vi "fake_scope.vi"() -> ()   [LabVIEW 2013]
doc: "This example shows how to use autosetup and acquire a waveform on a single channel for acquiring waveforms in a loop until stopped by user."
uses:
  osc_channel.ctl
  Global.vi
panel:
  out "SQUID":string="2"
  in  "stop":bool
  in  "Tab Control":T1(tab)
  out "Saving":bool
  out "Waveform Data":waveform(dbl)[](graph)=[{"t0"=timestamp(0 s since 1904-01-01), "dt"=6e-09, "Y"=array[1000 elements]}, {"t0"=timestamp(0 s since 1904-01-01), "dt"=6e-09, "Y"=array[1000 elements]}]
  in  "Points":i32=1000
  out "dt":dbl=6e-09 format="%#_2e"
  out "Repeat":u32=16
  out "Manufacturer":string="Skynet"
  out "Model":string="T1000"
  in  "Record":bool[](array[boolean])=[TRUE, FALSE]
  out "Stats":T2(array[cluster])=[{"Min"=-0.9973419383523257, "t (min)"=4.686e-06, "Max"=1.093351892163248, "t (max)"=1.53e-06, "Range"=2.0906938305155736, "Mean"=0.058141922470583494, "Std"=0.7227490723476767}, {"Min"=-0.5, "t (min)"=3.6779999999999998e-06, "Max"=0.5, "t (max)"=4.44e-07, "Range"=1.0, "Mean"=0.021262229190316277, "Std"=0.4513064444152934}] {"t (min)" format="%#_6p"; "t (max)" format="%#_6p"}
  in  "Channels":T3[](array[typedef])=[{"channel name"="CHANNEL1", "probe attenuation"=1.0, "vertical offset"=0.0, "vertical range"=10.0, "vertical coupling"=1, "input impedance"=50.0}, {"channel name"="CHANNEL2", "probe attenuation"=1.0, "vertical offset"=0.0, "vertical range"=1.0, "vertical coupling"=1, "input impedance"=50.0}] {"input impedance" format="%#_13g"; "vertical coupling" items=["AC", "DC", "GND"]; "vertical range" format="%.3f"; "vertical offset" format="%.3f"; "probe attenuation" format="%.3f"}
  in  "wait (ms)":u32=500
  in  "Bin size":i16=1
  in  "sample":dbl=6e-06
  in  "amplitude":dbl=1.0 format="%#_13g"
  in  "noise":dbl=0.1 format="%#_13g"
  in  "frequency":dbl=1000000.0 format="%#_13g"
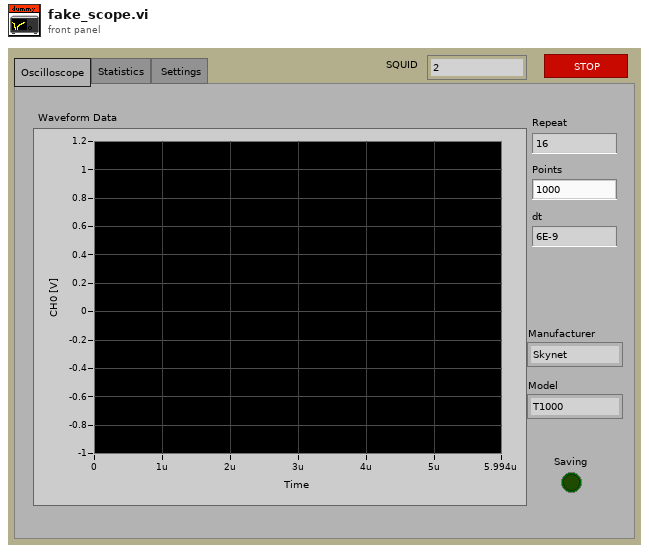
[diagram p1: front panel]
types:
  T1 = enum32{"Oscilloscope", "Statistics", " Settings"}
  T2 = cluster{"Min":dbl, "t (min)":dbl, "Max":dbl, "t (max)":dbl, "Range":dbl, "Mean":dbl, "Std":dbl}[]
  T3 = typedef "osc_channel.ctl" = cluster{"channel name":string, "probe attenuation":dbl, "vertical offset":dbl, "vertical range":dbl, "vertical coupling":i32, "input impedance":dbl}
  T4 = cluster{"Min":dbl, "t (min)":dbl, "Max":dbl, "t (max)":dbl, "Range":dbl, "Mean":dbl, "Std":dbl}
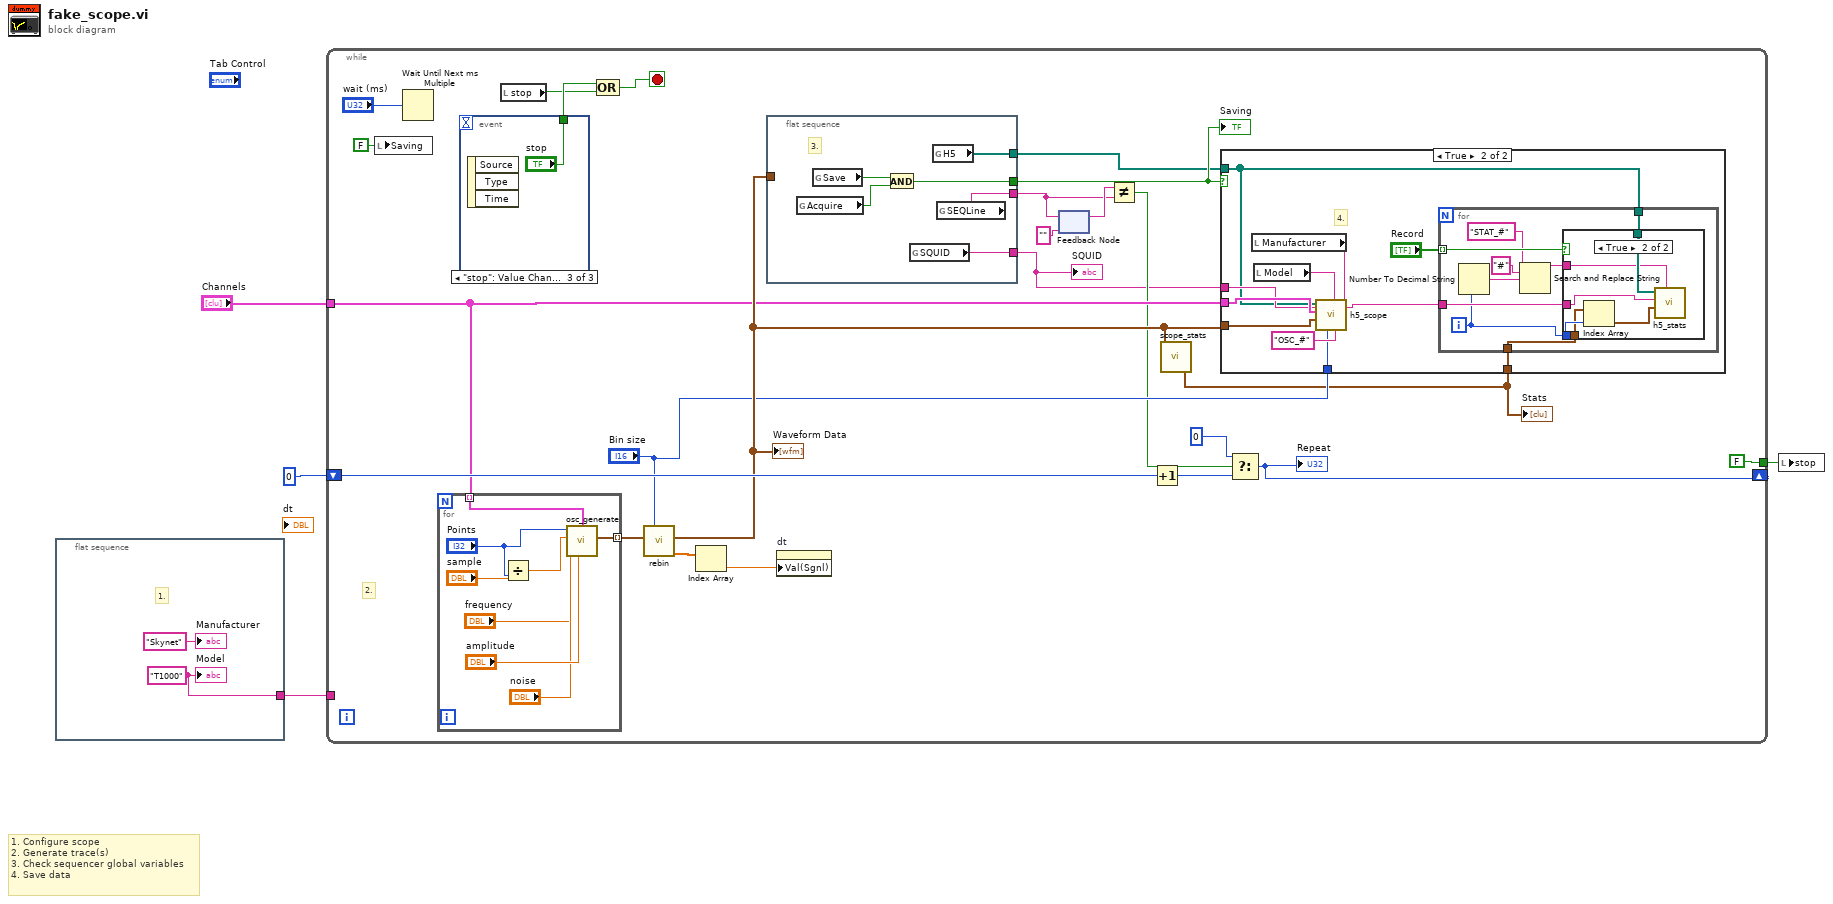
[diagram p0: block diagram]
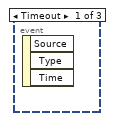
[diagram p4: hidden frame]
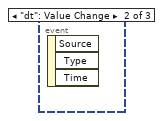
[diagram p5: hidden frame]
diagram:
  # "1. Configure scope\n2. Generate trace(s)\n3. Check sequencer global variables\n4. Save data"
  n1 = flat-sequence {
    tunnel: [w5] -> w1
    frame #0 {
      w5 = "T1000" ("Model")
      # "1."
      "Manufacturer" <- "Skynet" ("Manufacturer")
      "Model" <- w5
    }
  }
  n2 = while {
    shift-right: [w27] -> _
    shift-left: u32 0 ("millisecond multiple") -> [w28]
    tunnel: [FALSE ("stop")] -> w3
    tunnel: "Channels" -> [w17]
    tunnel: w1 -> [_]
    stop <- w29 stop-if-true
    # "2."
    n3 = local write "Saving"(FALSE ("Saving")) -> ()
    n4 = Wait Until Next ms Multiple(millisecond multiple="wait (ms)") -> ()  [unwired: 1 out]
    n5 = for {
      tunnel: [w69] -> w21 mode=indexing
      tunnel: w17 -> [w70] mode=indexing
      n6 = Divide(x="sample", y="Points") -> (x/y=w68:dbl)
      n7 = call "osc_generate.vi"("amplitude"="amplitude", "CHAN"=w70, "frequency"="frequency", "noise"="noise", "dt"=w68, "Points"="Points") -> ("output waveform"=w69:waveform(dbl))  [unwired: 5 in]
    }
    n8 = event shown="[2] \"stop\": Value Change" {
      selector: _ -> [_ _ _]
      dyn-events: _ -> [_ _ _]
      timeout: _ -> [_ _ _]
      tunnel: [_ _ "stop"] -> w25
      event Timeout {
        n9 = event-data() -> ()  [unwired: 1 in, 3 out]
      }
      event "dt": Value Change {
        n10 = event-data() -> ()  [unwired: 1 in, 3 out]
      }
      event "stop": Value Change {
        n11 = event-data() -> ()  [unwired: 1 in, 3 out]
      }
    }
    n12 = local read "stop"() -> (w24:bool)
    n13 = Compound Arithmetic op=OR(w25, w24) -> (w29:bool)
    n14 = call "rebin.vi"("Bin size"="Bin size", "Waveform Data IN"=w21) -> ("dt"=w19:dbl[], "Waveform Data OUT"=w22:waveform(dbl)[])  [unwired: 6 in, 1 out]
    "Waveform Data" <- w22
    n15 = Index Array(array=w19) -> (element=w20:dbl)  [unwired: 1 in]
    n16 = flat-sequence {
      tunnel: w22 -> [_]
      tunnel: [w34] -> w11
      tunnel: [w33] -> w10
      tunnel: [w32] -> w9
      tunnel: [w31] -> w8
      frame #0 {
        # "3."
        n17 = global read "Global.vi" "Acquire"() -> (w36:bool)
        n18 = global read "Global.vi" "Save"() -> (w35:bool)
        n19 = And(x=w35, y=w36) -> (x .and. y?=w34:bool)
        n20 = global read "Global.vi" "SQUID"() -> (w31:string)
        n21 = global read "Global.vi" "H5"() -> (w32:path[])
        n22 = global read "Global.vi" "SEQLine"() -> (w33:string)
      }
    }
    n23 = property on="dt" class="DigNum (strict)"("Val(Sgnl)"=w20) -> ()  [unwired: 2 in, 2 out]
    n24 = feedback #1("" ("Seq")) -> (w15:string)
    n25 = feedback-in #1(w10) -> ()
    n26 = Not Equal?(x=w15, y=w10) -> (x != y?=w12:bool)
    n27 = Increment(x=w28) -> (x+1=w13:u32)
    n28 = call "scope_stats.vi"("Waveform Data"=w22) -> ("Stats"=w7:T2)  [unwired: 7 in]
    "Stats" <- w7
    n29 = case shown="True" w11 {
      tunnel: w22 -> [_ w46]
      tunnel: w17 -> [_ w44]
      tunnel: w9 -> [_ w37]
      tunnel: w8 -> [_ w38]
      tunnel: "Bin size" -> [_ w41]
      tunnel: w7 -> [_ w39]
      frame False {
      }
      frame True {
        # "4."
        n30 = local read "Manufacturer"() -> (w43:string)
        n31 = local read "Model"() -> (w42:string)
        n32 = call "h5_scope.vi"("Model"=w42, "TYPE"="OSC_#", "Manufacturer"=w43, "Bin size"=w41, "SQUID"=w38, "Waveform Data"=w46, "Channels"=w44, "H5"=w37) -> ()  [unwired: 3 in, 1 out]
        n33 = for {
          tunnel: "Record" -> [w54] mode=indexing
          tunnel: w39 -> [w55]
          tunnel: w38 -> [w53]
          tunnel: w37 -> [w52]
          i -> [w50]
          n34 = Number To Decimal String(number=w50) -> (decimal integer string=w49:string)  [unwired: 1 in]
          n35 = Search and Replace String(input string="STAT_#", search string="#", replace string=w49) -> (result string=w48:string)  [unwired: 5 in, 3 out]
          n36 = case shown="True" w54 {
            tunnel: w50 -> [_ w61]
            tunnel: w55 -> [_ w60]
            tunnel: w53 -> [_ w58]
            tunnel: w52 -> [_ w57]
            tunnel: w48 -> [_ w56]
            frame False {
            }
            frame True {
              n37 = Index Array(array=w60, index=w61) -> (element=w59:T4)
              n38 = call "h5_stats.vi"("TYPE"=w56, "statistics"=w59, "SQUID"=w58, "H5"=w57) -> ()  [unwired: 6 in, 2 out]
            }
          }
        }
      }
    }
    n39 = Select(t=u32 0, s=w12, f=w13) -> (s? t:f=w27:u32)
    "Repeat" <- w27
    "Saving" <- w11
    "SQUID" <- w8
  }
  n40 = local write "stop"(w3) -> ()
